vi "Calculate Trigger Enable Phase Adjustment.vi"(9 "trigger enable period":u16, 10 "slave measurement":u16, 11 "master measurement":u16) -> (3 "trigger enable adjust amount":i32)   [LabVIEW 2011, in "FlexRIO Host Library (User).lvlib"]
uses:
  FlexRIO Host Library (User).lvlib
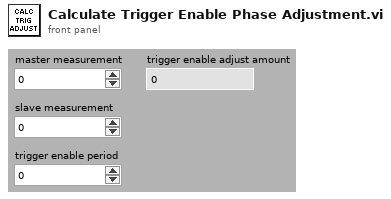
[diagram p1: front panel]
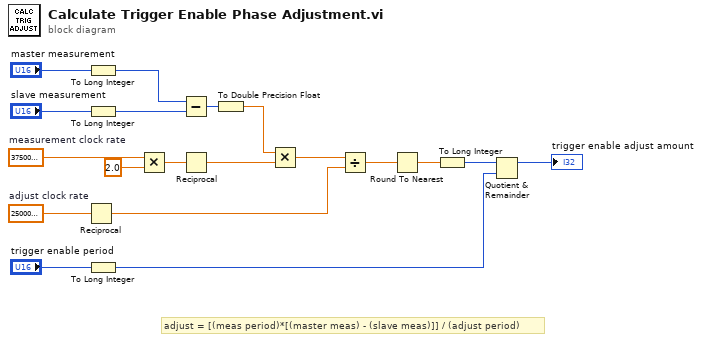
[diagram p0: block diagram]
diagram:
  w19 = 250000000.0  # adjust clock rate
  w10 = 375000000.0  # measurement clock rate
  # "adjust = [(meas period)*[(master meas) - (slave meas)]] / (adjust period)"
  n1 = Reciprocal(x=w19) -> (1/x=w14:dbl)
  n2 = To Long Integer(number="master measurement") -> (32bit integer=w7:i32)
  n3 = To Long Integer(number="slave measurement") -> (32bit integer=w6:i32)
  n4 = To Long Integer(number="trigger enable period") -> (32bit integer=w2:i32)
  n5 = Multiply(x=w10, y=2.0) -> (x*y=w11:dbl)
  n6 = Subtract(x=w7, y=w6) -> (x-y=w16:i32)
  n7 = Reciprocal(x=w11) -> (1/x=w4:dbl)
  n8 = To Double Precision Float(number=w16) -> (double precision float=w5:dbl)
  n9 = Multiply(x=w5, y=w4) -> (x*y=w15:dbl)
  n10 = Divide(x=w15, y=w14) -> (x/y=w13:dbl)
  n11 = Round To Nearest(number=w13) -> (nearest integer value=w12:dbl)
  n12 = To Long Integer(number=w12) -> (32bit integer=w3:i32)
  n13 = Quotient & Remainder(x=w3, y=w2) -> (x-y*floor(x/y)=→"trigger enable adjust amount":i32)  [unwired: 1 out]
